vi "Charger_Open Telemetry Session.vi"(6 "Stop Refnum":refnum<vi>, 7 "Status Refnum":T1, 8 "error in":errorcluster) -> (0 "error out":errorcluster, 2 "Ready":bool)   [LabVIEW 2020]
uses:
  Charger_Status Refnum.ctl
  Drivers/Charger Test Set/Charger_Input Control.ctl
  Drivers/Telemetry/Typedef Command List.ctl
panel:
  in  "F_msg":string="Failed to establish Telemetry session."
  in  "P_msg":string="Telemetry session open."
  in  "fmt":string="Opening Telemetry session for MICS ID 0x%4x."
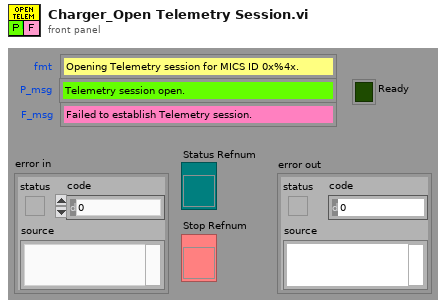
[diagram p1: front panel]
types:
  T1 = typedef "Charger_Status Refnum.ctl" = refnum<vi>
  T2 = typedef "Typedef Command List.ctl" = enum16{"Get xPG Status", "xPG Stimulation", "Select Program", "Increment Program Amplitude", "Decrement Program Amplitude", "Get PoP Constants", "Get PPC Constants", "Get Program Names", "Set Pulse Amplitude", "Increment Pulse Amplitude", "Decrement Pulse Amplitude", "Get Pulse Widths", "Set Pulse Widths", "Increment Pulse Width", "Decrement Pulse Width", "Get Program Frequency", "Set Program Frequency", "Increment Program Frequency", "Decrement Program Frequency", "Inject Event", "Charging Control", "Get xPG Identity", "Set xPG Identity", "Restore Program Defaults", "Get Program Definition", "Set Program Definition", "Get Program Constants", "Set Program Constants", "Get Configurable Device Parameters", "Set Configurable Device Parameters", "Get Pulse Constants", "Set Pulse Constants", "Get Lead Limits", "Set Lead Limits", "Get Channel Calibrations", "Set Channel Calibrations", "<reserved 2>", "<reserved 3>", "<reserved 4>", "<reserved 5>", "<reserved 6>", "<reserved 7>", "Get Stim Asic HV Calibrations", "Set Stim Asic HV Calibrations", "<reserved 8>", "<reserved 9>", "Get CP Data", "Set CP Data", "Clear Log", "Read Log", "Append Log", "Get Patient Program Runtime", "Set Patient Program Runtime", "Impedance Measurement", "Enter Storage Mode", "Echo Short", "Echo Long", "Get General Calibration", "Set General Calibration", "Get Trim List", "Set Trim List", "Get Counter", "Set Counter", "Get Test Stimulation", "Set Test Stimulation", "Get Titration Stimulation", "Set Titration Stimulation", "Get Ramp Time", "Set Ramp Time", "Get VBAT", "Set Software Description Block", "Get Software Description Block", "Write Memory", "Read Memory", "Reset xPG", "Erase Flash Block", "Write Vectors", "Read Vectors", "Diagnostic Data", "Set Background Impedance", "Get Background Impedence ", "Set Test Waveform", "Calibrate Channel", "Get Log Range", "Reserved 0x55", "Reserved 0x56", "MICS Options", "Pair PPC", "Pair POP", "Stop Bootloader", "Tune MICS", "MICS Diagnostics", "Undefined"}
  T3 = cluster{"Command":T2, "Function":enum16{"Open Session", "Close Session", "Downlink Only", "Uplink Only", "Transceive (DN -> UP)"}, "MICS_ID":u32, "EXID":u32, "Use Local":bool, "Transceive Delay mS":dbl, "CP_DATA IN":u8[], "Parameters":string}
  T4 = typedef "MICS_Input Control.ctl" = cluster{"address":refnum<visa-resource-name>, "chan":u16, "ID":u32}
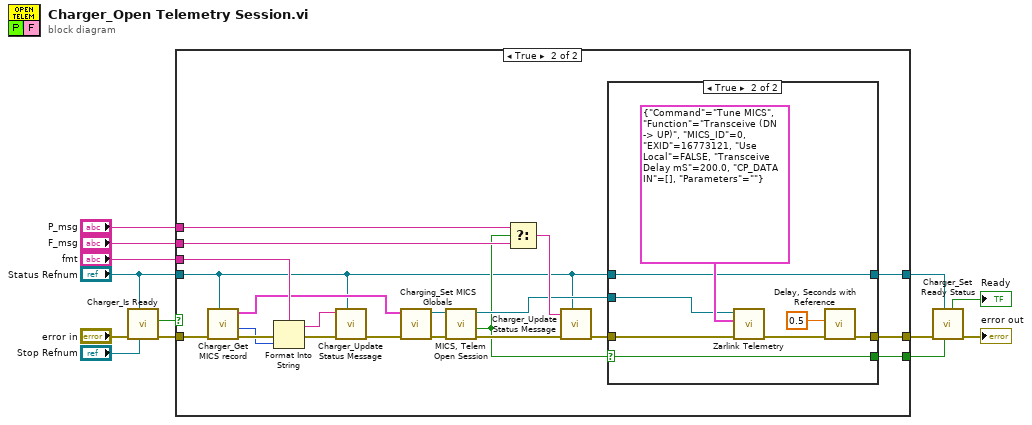
[diagram p0: block diagram]
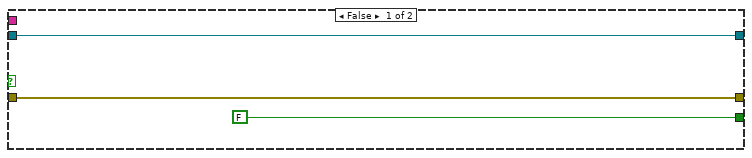
[diagram p2: hidden frame]
diagram:
  n1 = call "Charger_Is Ready.vi"("Stop Refnum"="Stop Refnum", "Status Refnum"="Status Refnum", "error in"="error in") -> ("error out"=w11:errorcluster, "ready"=w10:bool)  [unwired: 7 in]
  n2 = case shown="True" w10 {
    tunnel: [w16 w21] -> w4
    tunnel: "Status Refnum" -> [w14 w19]
    tunnel: w11 -> [w16 w26]
    tunnel: "fmt" -> [_ w28]
    tunnel: "P_msg" -> [_ w32]
    tunnel: "F_msg" -> [_ w31]
    tunnel: [FALSE ("in_session") w17] -> w3
    tunnel: [w14 w18] -> w2
    frame False {
    }
    frame True {
      n3 = call "Charger_Get MICS record.vi"("Status Refnum"=w19, "error in"=w26) -> ("error out"=w27:errorcluster, "ID"=w25:u32, "MICS Inputs"=w24:T4)  [unwired: 3 in, 2 out]
      n4 = Format Into String(format string=w28, error in=w27, w25) -> (resulting string=w29:string, error out=w30:errorcluster)  [unwired: 1 in]
      n5 = call "Charger_Update Status Message.vi"("Status Refnum"=w19, "error in"=w30, "status message"=w29) -> ("error out"=w35:errorcluster)  [unwired: 6 in]
      n6 = call "Charging_Set MICS Globals.vi"("error in"=w35, "MICS inputs"=w24) -> ("error out"=w37:errorcluster, "address"=w36:refnum<visa-resource-name>)  [unwired: 4 in]
      n7 = call "MICS, Telem Open Session.vi"("error in"=w37, "VISA resource"=w36) -> ("error out"=w34:errorcluster, "in_session"=w20:bool, "VISA resource dup"=w22:refnum<visa-resource-name>)  [unwired: 7 in]
      n8 = Select(t=w32, s=w20, f=w31) -> (s? t:f=w33:string)
      n9 = call "Charger_Update Status Message.vi"("Status Refnum"=w19, "error in"=w34, "status message"=w33) -> ("error out"=w23:errorcluster)  [unwired: 6 in]
      n10 = case shown="True" w20 {
        selector: w20 -> [w39 w41]
        tunnel: w23 -> [w40 w47]
        tunnel: w22 -> [_ w46]
        tunnel: [w40 w44] -> w21
        tunnel: w19 -> [w38 w42]
        tunnel: [w38 w42] -> w18
        tunnel: [w39 w41] -> w17
        frame False {
        }
        frame True {
          n11 = call "Zarlink Telemetry.vi"("error in (no error)"=w47, "Input"=T3 {"Command"=enum."Tune MICS", "Function"=enum."Transceive (DN -> UP)", "MICS_ID"=0, "EXID"=16773121, "Use Local"=FALSE, "Transceive Delay mS"=200.0, "CP_DATA IN"=[], "Parameters"=""}, "MICS Dongle Address"=w46) -> ("error out"=w45:errorcluster)  [unwired: 6 in, 2 out]
          n12 = call "Delay, Seconds with Reference.vi"("error in"=w45, "delay"=dbl[unit] 0.5) -> ("error out"=w44:errorcluster)  [unwired: 4 in, 2 out]
        }
      }
    }
  }
  n13 = call "Charger_Set Ready Status.vi"("Ready"=w3, "Status Refnum"=w2, "error in"=w4) -> ("error out"=→"error out":errorcluster, "Ready Status"=→"Ready":bool)  [unwired: 6 in]
